vi "MQTT_Read_Anything.vi"() -> ()   [LabVIEW 2012, in "MQTT_Functions.lvlib"]
uses:
  MQTT_Functions.lvlib
  Controls/MessageType.ctl
panel:
  out "Message ID":u16=1 format="%x"
  out "Topic Name":string="Topic"
  out "Message":string="MQIsdp"
  out "MessageType":T1
  out "connection ID out":refnum<k5>
  in  "connection ID":refnum<k5>
  out "error out":errorcluster
  in  "error in (no error)":errorcluster
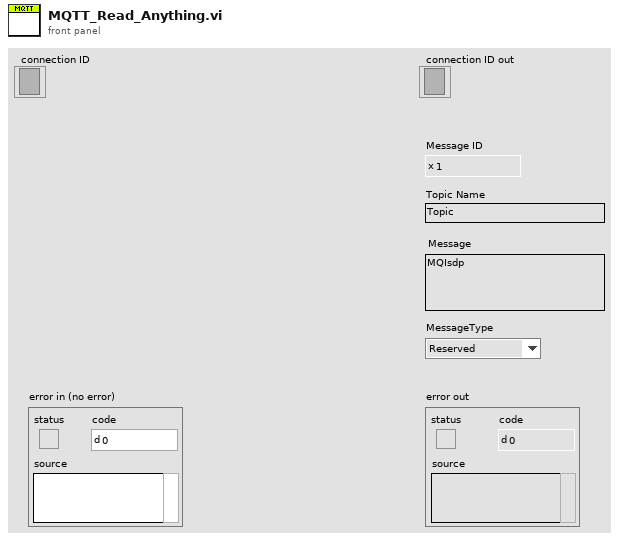
[diagram p1: front panel]
types:
  T1 = typedef "MQTT_Functions.lvlib/MessageType.ctl" = enum32{"Reserved", "CONNECT", "CONNACK", "PUBLISH", "PUBACK", "PUBREC", "PUBREL", "PUBCOMP", "SUBSCRIBE", "SUBACK", "UNSUBSCRIBE", "UNSUBACK", "PINGREQ", "PINGRESP", "DISCONNECT", "Reserved2"}
  T2 = typedef "MQTT_Functions.lvlib/QoS.ctl" = enum8{"At most once", "At least once", "Exactly once", "Reserved"}
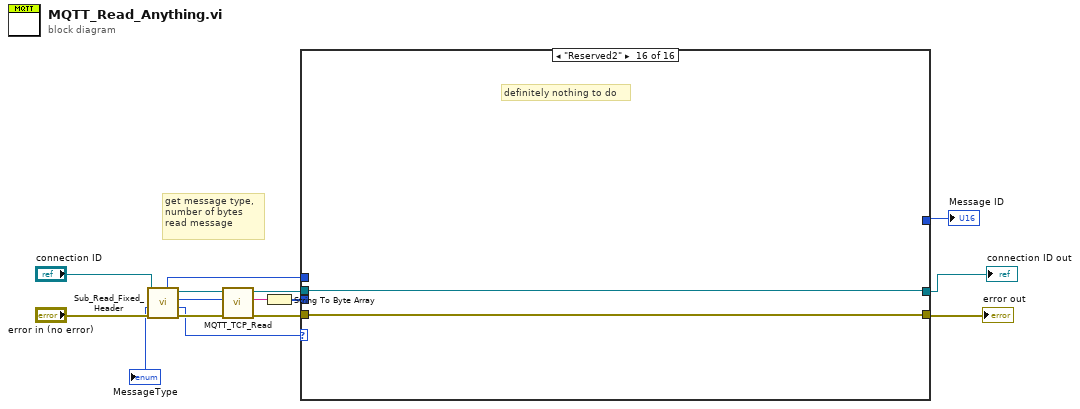
[diagram p0: block diagram]
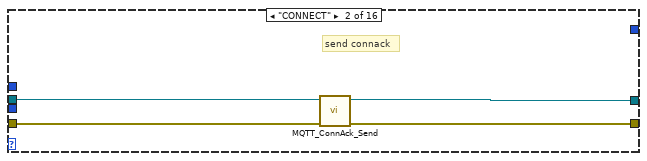
[diagram p3: hidden frame]
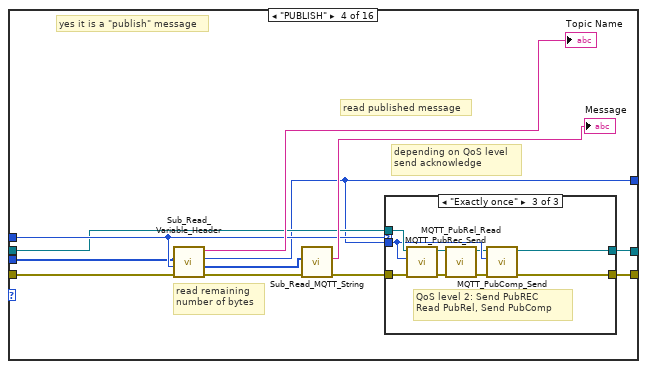
[diagram p5: hidden frame]
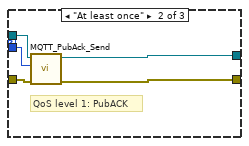
[diagram p7: hidden frame]
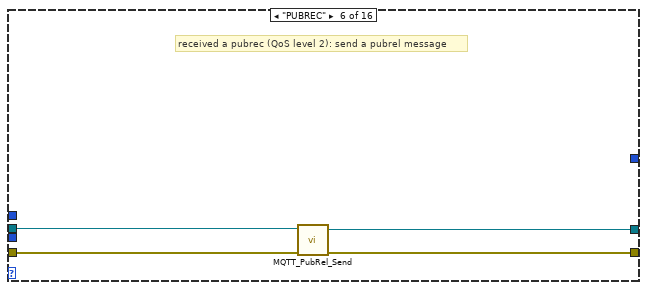
[diagram p9: hidden frame]
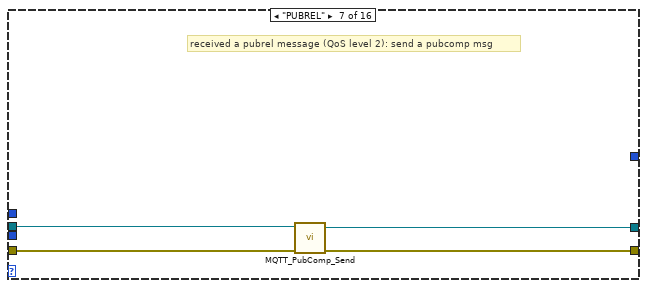
[diagram p10: hidden frame]
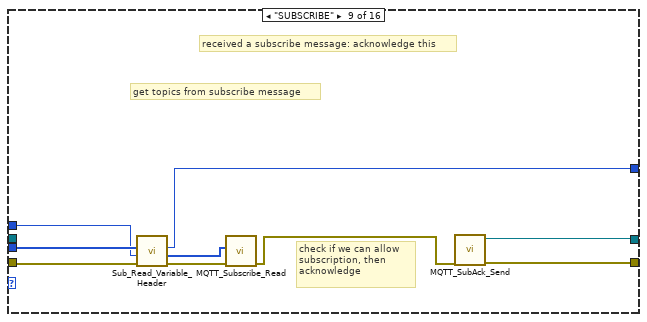
[diagram p12: hidden frame]
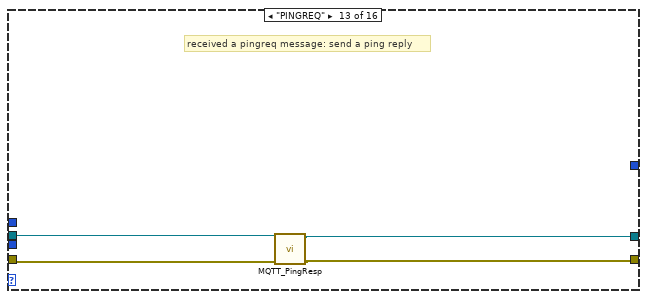
[diagram p16: hidden frame]
diagram:
  # "get message type, \nnumber of bytes\nread message"
  n1 = call "Sub_Read_Fixed_Header.vi"("error in (no error)"="error in (no error)", "connection ID"="connection ID") -> ("error out"=w8:errorcluster, "MessageType"=w3:T1, "Remaining Length"=w9:u32, "connection ID out"=w7:refnum<k5>, "QoS Level"=w11:T2)  [unwired: 3 in, 2 out]
  "MessageType" <- w3
  n2 = call "MQTT_TCP_Read.vi"("error in (no error)"=w8, "bytes to read"=w9, "connection ID"=w7) -> ("error out"=w5:errorcluster, "data out"=w4:string, "connection ID out"=w6:refnum<k5>)  [unwired: 6 in]
  n3 = String To Byte Array(string=w4) -> (unsigned byte array=w2:u8[])
  n4 = case shown="\"Reserved2\"" w3 {
    tunnel: w5 -> [w16 w20 w22 w26 w52 w56 w60 w62 w69 w73 w75 w77 w81 w83 w85 w87]
    tunnel: [w16 w17 w22 w27 w52 w55 w59 w62 w71 w73 w75 w77 w78 w83 w85 w87] -> w13
    tunnel: w11 -> [_ _ _ w29 _ _ _ _ w66 _ _ _ _ _ _ _]
    tunnel: w6 -> [w15 w19 w21 w25 w51 w53 w58 w61 _ w72 w74 w76 w80 w82 w84 w86]
    tunnel: [w15 w18 w21 w28 w51 w54 w57 w61 w70 w72 w74 w76 w79 w82 w84 w86] -> w10
    tunnel: w2 -> [_ _ _ w24 _ _ _ _ w68 _ _ _ _ _ _ _]
    tunnel: [_ _ _ w23 _ _ _ _ w67 _ _ _ _ _ _ _] -> w1
    frame "Reserved", Default {
    }
    frame "CONNECT" {
      # "send connack"
      n5 = call "MQTT_ConnAck_Send.vi"("error in (no error)"=w20, "connection ID"=w19) -> ("error out"=w17:errorcluster, "connection ID out"=w18:refnum<k5>)  [unwired: 7 in, 1 out]
    }
    frame "CONNACK" {
      # "connection was acknowledged: nothing to do"
    }
    frame "PUBLISH" {
      # "yes it is a \"publish\" message"
      # "depending on QoS level\nsend acknowledge"
      # "read remaining\nnumber of bytes"
      # "read published message"
      n6 = call "Sub_Read_Variable_Header.vi"("error in (no error)"=w26, "QoS"=w29, "Variable Header"=w24) -> ("error out"=w33:errorcluster, "remaining bytes"=w31:u8[], "Message ID"=w23:u16, "Topic Name"=→"Topic Name":string)  [unwired: 5 in]
      n7 = call "Sub_Read_MQTT_String.vi"("error in (no error)"=w33, "UTF8 Byte Array"=w31) -> ("error out"=w30:errorcluster, "String"=→"Message":string)  [unwired: 7 in, 1 out]
      n8 = case shown="\"Exactly once\"" w29 {
        tunnel: w23 -> [_ w41 w46]
        tunnel: w30 -> [w35 w40 w50]
        tunnel: w25 -> [w36 w39 w49]
        tunnel: [w36 w38 w48] -> w28
        tunnel: [w35 w37 w47] -> w27
        frame "At most once", Default {
          # "QoS level 0, no ACK"
        }
        frame "At least once" {
          # "QoS level 1: PubACK"
          n9 = call "MQTT_PubAck_Send.vi"("error in (no error)"=w40, "Message ID"=w41, "connection ID"=w39) -> ("error out"=w37:errorcluster, "connection ID out"=w38:refnum<k5>)  [unwired: 6 in, 1 out]
        }
        frame "Exactly once" {
          # "QoS level 2: Send PubREC\nRead PubRel, Send PubComp"
          n10 = call "MQTT_PubRec_Send.vi"("error in (no error)"=w50, "Message ID"=w46, "connection ID"=w49) -> ("error out"=w43:errorcluster, "connection ID out"=w42:refnum<k5>)  [unwired: 6 in, 1 out]
          n11 = call "MQTT_PubRel_Read.vi"("error in (no error)"=w43, "connection ID"=w42) -> ("error out"=w44:errorcluster, "connection ID out"=w45:refnum<k5>)  [unwired: 7 in, 1 out]
          n12 = call "MQTT_PubComp_Send.vi"("error in (no error)"=w44, "Message ID"=w46, "connection ID"=w45) -> ("error out"=w47:errorcluster, "connection ID out"=w48:refnum<k5>)  [unwired: 6 in, 1 out]
        }
      }
    }
    frame "PUBACK" {
      # "read puback"
      # "received a puback (QoS level 1): nothing to do!"
    }
    frame "PUBREC" {
      # "received a pubrec (QoS level 2): send a pubrel message"
      n13 = call "MQTT_PubRel_Send.vi"("error in (no error)"=w56, "connection ID"=w53) -> ("error out"=w55:errorcluster, "connection ID out"=w54:refnum<k5>)  [unwired: 7 in, 1 out]
    }
    frame "PUBREL" {
      # "received a pubrel message (QoS level 2): send a pubcomp msg"
      n14 = call "MQTT_PubComp_Send.vi"("error in (no error)"=w60, "connection ID"=w58) -> ("error out"=w59:errorcluster, "connection ID out"=w57:refnum<k5>)  [unwired: 7 in, 1 out]
    }
    frame "PUBCOMP" {
      # "received a pubcomp message (QoS level 2): nothing to do"
    }
    frame "SUBSCRIBE" {
      # "check if we can allow \nsubscription, then \nacknowledge"
      # "get topics from subscribe message"
      # "received a subscribe message: acknowledge this"
      n15 = call "Sub_Read_Variable_Header.vi"("error in (no error)"=w69, "QoS"=w66, "Variable Header"=w68) -> ("error out"=w64:errorcluster, "remaining bytes"=w65:u8[], "Message ID"=w67:u16)  [unwired: 5 in, 1 out]
      n16 = call "MQTT_Subscribe_Read.vi"("error in (no error)"=w64, "Bytes Read"=w65) -> ("error out"=w63:errorcluster)  [unwired: 8 in, 1 out]
      n17 = call "MQTT_SubAck_Send.vi"("error in (no error)"=w63) -> ("error out"=w71:errorcluster, "connection ID out"=w70:refnum<k5>)  [unwired: 8 in, 1 out]
    }
    frame "SUBACK" {
      # "received suback from server. nothing to do"
    }
    frame "UNSUBSCRIBE" {
      # "received an unsubscribe message: unsubscribe from selected topics"
    }
    frame "UNSUBACK" {
      # "received unsuback message: nothing to do"
    }
    frame "PINGREQ" {
      # "received a pingreq message: send a ping reply"
      n18 = call "MQTT_PingResp.vi"("error in (no error)"=w81, "connection ID"=w80) -> ("error out"=w78:errorcluster, "connection ID out"=w79:refnum<k5>)  [unwired: 7 in, 1 out]
    }
    frame "PINGRESP" {
      # "received a ping response: server is alive"
    }
    frame "DISCONNECT" {
      # "received a disconnect signal"
    }
    frame "Reserved2" {
      # "definitely nothing to do"
    }
  }
  "error out" <- w13
  "connection ID out" <- w10
  "Message ID" <- w1
